vi "실습 10-6.vi"() -> ()   [LabVIEW 2014]
uses:
  <vilib>/addons/database/Connection.llb/DB Tools Open Connec (Path).vi
  <vilib>/addons/database/Connection.llb/Conn Execute.vi
  <vilib>/addons/database/Recordset.llb/Rec Fetch Recordset Data (R).vi
  <vilib>/addons/database/Recordset.llb/Rec Destroy - Connection.vi
  <vilib>/addons/database/NI_Database_API.lvlib
panel:
  out "데이터":i32[](array[numeric])
  out "recordset data":variant[][](array[variant])
  in  "SQL query":string
  in  "경로":path
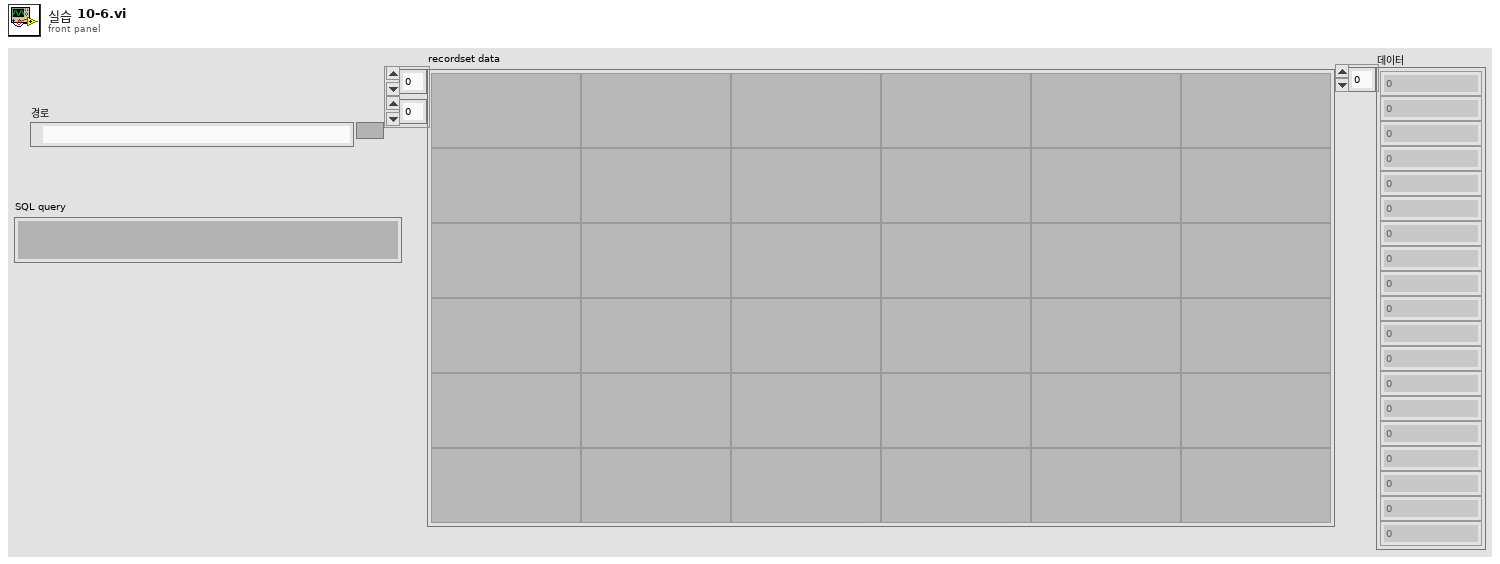
[diagram p1: front panel]
types:
  T1 = typedef "NI_Database_API.lvlib/Conn ObjectReference.ctl" = refnum<k1>
  T2 = typedef "NI_Database_API.lvlib/Rec ObjectReference.ctl" = refnum<k1>
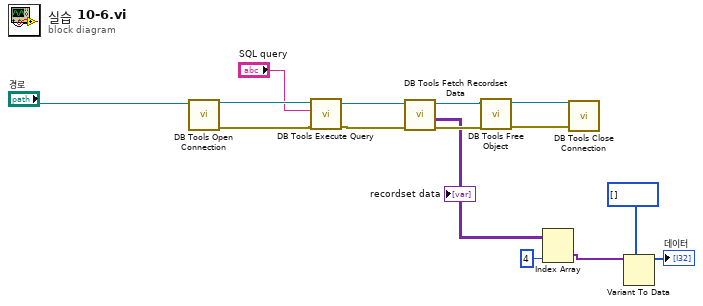
[diagram p0: block diagram]
diagram:
  n1 = call-poly <vilib>:"DB Tools Open Connection.vi"("connection information"="경로") -> ("error out"=w13:errorcluster, "connection reference"=w14:T1)  [unwired: 7 in]
  n2 = call-poly <vilib>:"DB Tools Execute Query.vi"("error in (no error)"=w13, "SQL query"="SQL query", "connection reference"=w14) -> ("error out"=w7:errorcluster, "recordset reference"=w9:T2)  [unwired: 5 in]
  n3 = call-poly <vilib>:"DB Tools Fetch Recordset Data.vi"("error in (no error)"=w7, "recordset reference"=w9) -> ("error out"=w6:errorcluster, "recordset data"=w5:variant[][], "recordset reference out"=w8:T2)  [unwired: 3 in]
  "recordset data" <- w5
  n4 = call-poly <vilib>:"DB Tools Free Object.vi"("error in (no error)"=w6, "recordset reference"=w8) -> ("error out"=w11:errorcluster, "connection reference"=w12:T1)  [unwired: 8 in]
  n5 = Index Array(array=w5, index (col)=4 ("비활성화된 인덱스 (열)")) -> (element=w3:variant[])  [unwired: 1 in]
  n6 = call <vilib>:"DB Tools Close Connection.vi"("error in (no error)"=w11, "connection reference"=w12) -> ()  [unwired: 5 in, 1 out]
  n7 = Variant To Data(type=i32[] [], Variant=w3) -> (data=→"데이터":i32[])  [unwired: 1 in, 1 out]
